vi "send-email-v5.vi"(10 "Message":string, 11 "Recipient emails":string[](array[string])) -> (0 "error out":errorcluster)   [LabVIEW 2019]
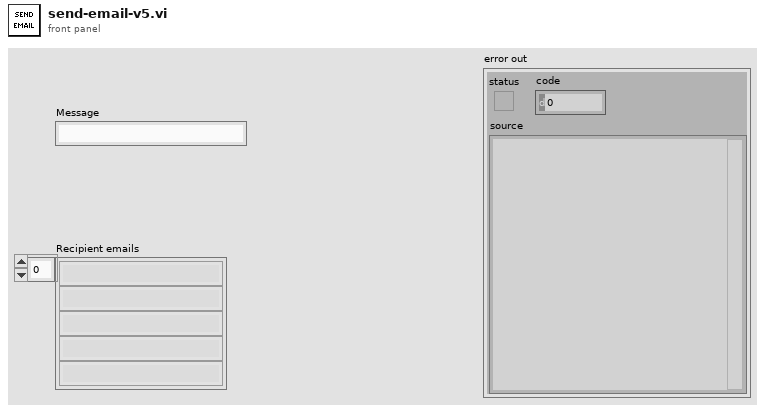
[diagram p1: front panel]
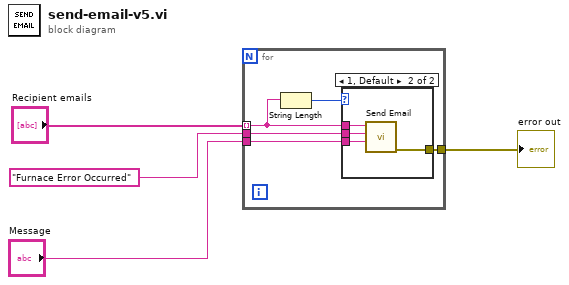
[diagram p0: block diagram]
diagram:
  n1 = for {
    tunnel: "Recipient emails" -> [w6] mode=indexing
    tunnel: "Message" -> [w9]
    tunnel: "Furnace Error Occurred" ("Subject") -> [w8]
    tunnel: [w7] -> w2
    n2 = String Length(string=w6) -> (length=w5:i32)
    n3 = case shown="1, Default" w5 {
      tunnel: w9 -> [_ w13]
      tunnel: w8 -> [_ w12]
      tunnel: [_ w11] -> w7
      tunnel: w6 -> [_ w10]
      frame 0 {
      }
      frame 1, Default {
        n4 = call "Send Email"("Message"=w13, "Subject"=w12, "Recipients"=w10) -> ("error out"=w11:errorcluster)  [unwired: 8 in]
      }
    }
  }
  "error out" <- w2
